vi "getDoppler_callDLL.vi"(6 "B scan period":dbl, 7 "FFTW3 Properties":T1={"data_points"=300, "camera_pixel"=2048, "zero array"=[], "complex zero array"=[]}, 8 "Error in":errorcluster, 9 "Spectrometer.lvclass":refnum<class "Spectrometer.lvclass">, 10 "Processing Settings":refnum<class "ConfigProc.lvclass">, 11 "Data_complex":dbl[][](array[numeric])) -> (0 "error out":errorcluster, 3 "velocity_profile":dbl[][](graph))   [LabVIEW 2017]
uses:
  classes/HardwareObjects/Spectrometer/Spectrometer.lvclass
  classes/SoftwareObjects/ConfigProc/ConfigProc.lvclass
  classes/HardwareObjects/Spectrometer/Spectrometer.lvclass/Spectrometer.ctl
  classes/SoftwareObjects/ConfigProc/ConfigProc.lvclass/ConfigProc.ctl
  classes/SoftwareObjects/ConfigProc/Read Cores.vi
  classes/HardwareObjects/Spectrometer/Read Center wavelength (nm).vi
  C/SD_OCT_DLL_Ver3/x64/Release/SD_OCT_DLL_Ver3.dll
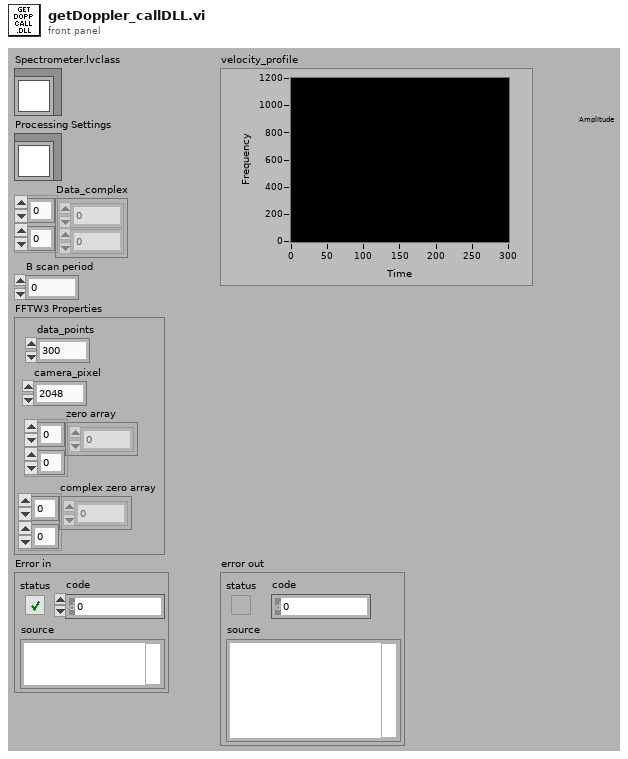
[diagram p1: front panel]
types:
  T1 = cluster{"data_points":i32, "camera_pixel":i32, "zero array":dbl[][], "complex zero array":dbl[][]}
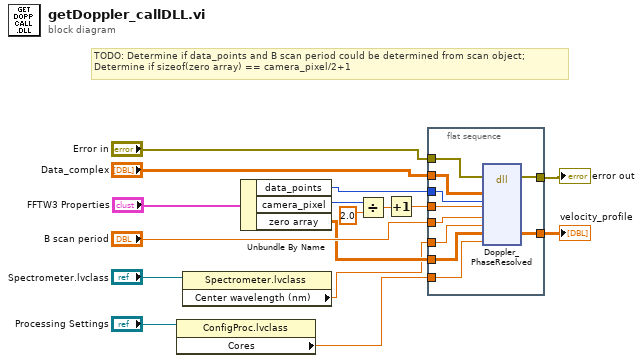
[diagram p0: block diagram]
diagram:
  # "TODO: Determine if data_points and B scan period could be determined from scan object;\nDetermine if sizeof(zero array) == camera_pixel/2+1"
  n1 = property class="ConfigProc.lvclass"(reference="Processing Settings") -> ("Cores"=w1:dbl)  [unwired: 1 in, 2 out]
  n2 = property class="Spectrometer.lvclass"(reference="Spectrometer.lvclass") -> ("Center wavelength (nm)"=w3:dbl)  [unwired: 1 in, 2 out]
  n3 = Unbundle By Name("FFTW3 Properties") -> ("data_points"=w11:i32, "camera_pixel"=w7:i32, "zero array"=w10:dbl[][])
  n4 = Divide(x=w7, y=2.0) -> (x/y=w6:dbl)
  n5 = Increment(x=w6) -> (x+1=w5:dbl)
  n6 = flat-sequence {
    tunnel: [w26] -> w16
    tunnel: "Error in" -> [w25]
    tunnel: "Data_complex" -> [w24]
    tunnel: w11 -> [w23]
    tunnel: "B scan period" -> [w22]
    tunnel: w3 -> [w17]
    tunnel: [w21] -> w12
    tunnel: w1 -> [w20]
    tunnel: w10 -> [w19]
    tunnel: w5 -> [w18]
    frame #0 {
      n7 = dll-call lib="F:/OCT-software/animal-octa/main/C/SD_OCT_DLL_Ver3/x64/Release/SD_OCT_DLL_Ver3.dll" fn="Doppler_PhaseResolved"(error in=w25, "Data_complex"=w24, "data_points"=w23, "camera_pixel"=w18, "period"=w22, "lambda"=w17, "velocity_profile"=w19, "core_number"=w20) -> (error out=w26:errorcluster, "velocity_profile"=w21:dbl[][])  [unwired: 9 in, 1 out]
    }
  }
  "error out" <- w16
  "velocity_profile" <- w12
